vi "change_connect_button_state.vi"(8 "error in (no error)":errorcluster, 10 "button_status":T1(ring), 11 "Boolean in":refnum<vi>) -> (0 "error out":errorcluster, 3 "Boolean out":refnum<vi>)   [LabVIEW 2018]
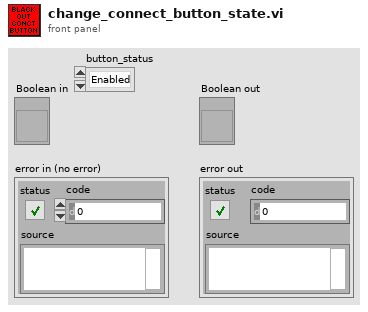
[diagram p1: front panel]
types:
  T1 = enum8{"Enabled", "Disabled", "Disabled and Grayed Out"}
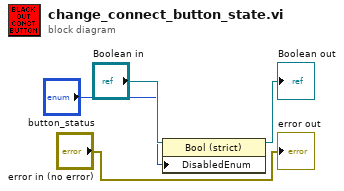
[diagram p0: block diagram]
diagram:
  n1 = property class="Bool (strict)"(reference="Boolean in", "DisabledEnum"="button_status") -> (reference out=→"Boolean out":refnum<vi>)  [unwired: 1 in, 1 out]
  "error out" <- "error in (no error)"
